vi "Frame IO to String.vi"(1 "Frame list":refnum<k21>[](array[refnum])) -> (0 "Frame list":string[](array[string]))   [LabVIEW 2021, in "BS120x Driver.lvlib" / "XNET_BS120x.lvclass"]
uses:
  XNET_BS120x.lvclass
  XNET_BS120x.lvclass/XNET_BS120x.ctl
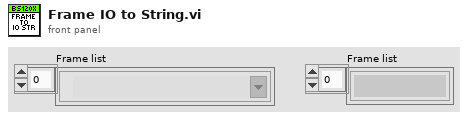
[diagram p1: front panel]
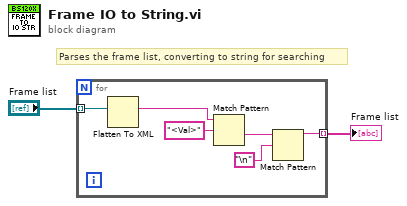
[diagram p0: block diagram]
diagram:
  # "Parses the frame list, converting to string for searching"
  n1 = for {
    tunnel: "Frame list" -> [w8] mode=indexing
    tunnel: [w3] -> w2 mode=indexing
    n2 = Flatten To XML(6:w8) -> (2:w5:string)
    n3 = Match Pattern(string=w5, regular expression="<Val>") -> (after substring=w4:string)  [unwired: 1 in, 3 out]
    n4 = Match Pattern(string=w4, regular expression="\n") -> (before substring=w3:string)  [unwired: 1 in, 3 out]
  }
  "Frame list" <- w2
